vi "comm options.vi"(8 "error in (no error)":errorcluster, 10 "options string":string, 11 "Comm Handle":u64) -> (0 "error out":errorcluster, 3 "dup Comm Handle":u64)   [LabVIEW 2009, in "lvserial.lvlib"]
doc: "Sets the serial port options. This function is also called inside the CommOpen function and allows the user to specify the major settings together with the serial port name in one string."
uses:
  lvserial.lvlib
  x64/Release/lvserial.dll
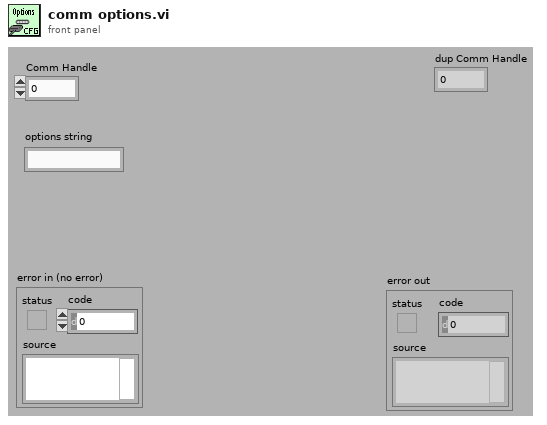
[diagram p1: front panel]
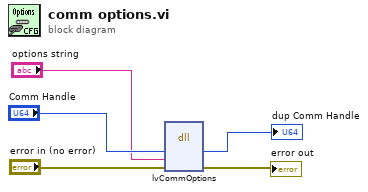
[diagram p0: block diagram]
diagram:
  n1 = dll-call lib="C:/Users/Admin/Desktop/lvserial_source_1-2-13/x64/Release/lvserial.dll" fn="lvCommOptions"("hComm"="Comm Handle", "shOptions"="options string", "pError"="error in (no error)") -> ("hComm"=→"dup Comm Handle":u64, "pError"=→"error out":errorcluster)  [unwired: 4 in, 3 out]
